vi "Cartesian To Complex.vi"   [LabVIEW 2017, in "NI_Matrix.lvlib"]
doc: "Creates a complex number from two values in rectangular notation."
uses:
  <vilib>/Analysis/Matrix/NI_Matrix.lvlib
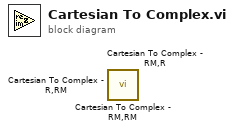
[diagram p0: block diagram]
diagram:
  n1 = call <vilib>:"Cartesian To Complex - RM,RM.vi"() -> ()  [unwired: 2 in, 1 out]
  n2 = call <vilib>:"Cartesian To Complex - RM,R.vi"() -> ()  [unwired: 2 in, 1 out]
  n3 = call <vilib>:"Cartesian To Complex - R,RM.vi"() -> ()  [unwired: 2 in, 1 out]
